vi "File_IO_Sample.vi"() -> ()   [LabVIEW 2025]
panel:
  out "Array 10":string[][](array[string])
  out "error out 2":errorcluster
  out "String 3":string
  out "Table Control":string[][](table)
  in  "Path":path
  out "error out":errorcluster
  in  "error in (no error)":errorcluster
  out "String 2":string
  in  "file path":path
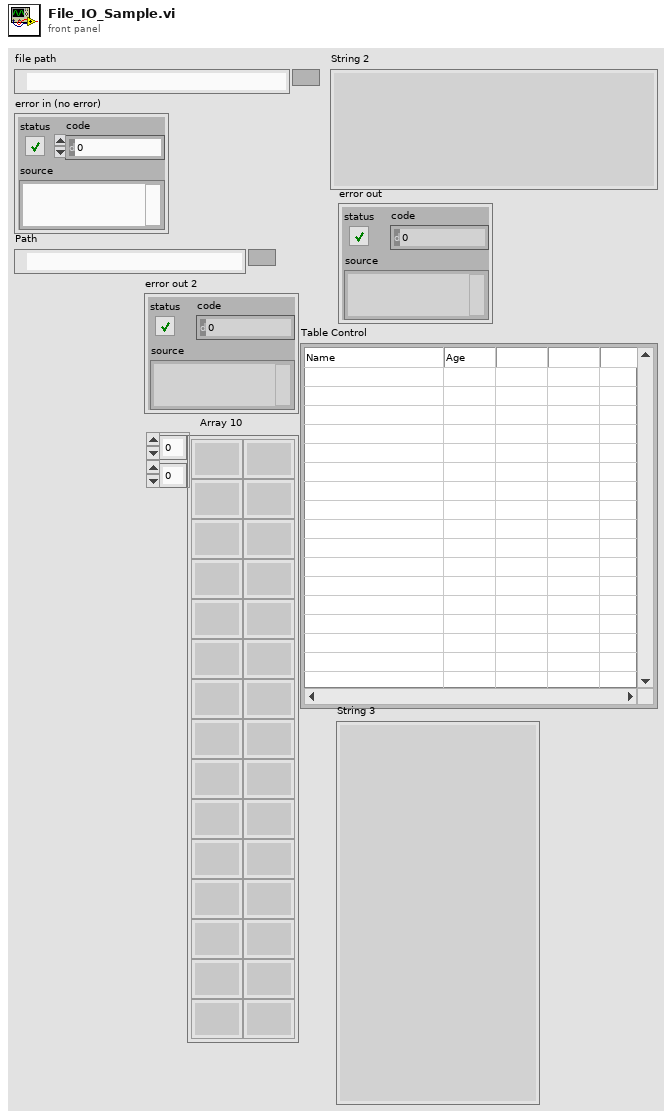
[diagram p1: front panel]
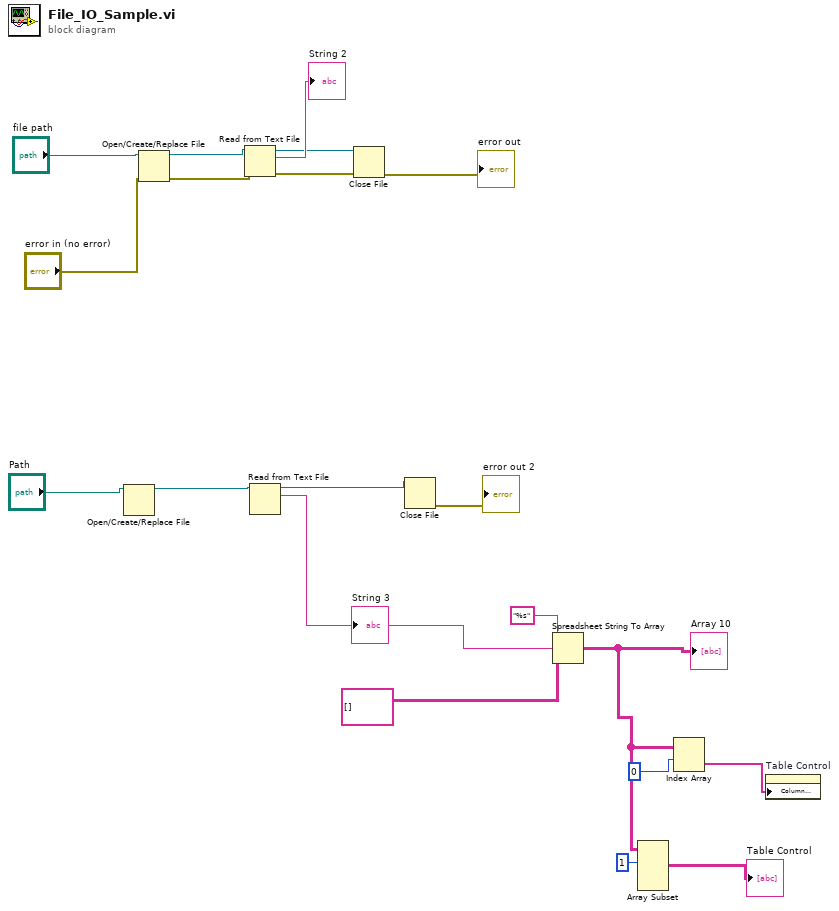
[diagram p0: block diagram]
diagram:
  n1 = Open/Create/Replace File(file path (use dialog)="Path") -> (refnum out=w11:refnum<file>)  [unwired: 5 in, 2 out]
  n2 = Open/Create/Replace File(file path (use dialog)="file path", error in="error in (no error)") -> (refnum out=w18:refnum<file>, error out=w17:errorcluster)  [unwired: 4 in, 1 out]
  n3 = Read from Text File(file (use dialog)=w18, error in=w17) -> (refnum out=w13:refnum<file>, text=→"String 2":string, error out=w15:errorcluster)  [unwired: 2 in, 1 out]
  n4 = Read from Text File(file (use dialog)=w11) -> (refnum out=w10:refnum<file>, text=w8:string)  [unwired: 3 in, 2 out]
  "String 3" <- w8
  n5 = Close File(refnum=w13, error in=w15) -> (error out=→"error out":errorcluster)  [unwired: 1 out]
  n6 = Close File(refnum=w10) -> (error out=→"error out 2":errorcluster)  [unwired: 1 in, 1 out]
  n7 = Spreadsheet String To Array(format string="%s", spreadsheet string=w8, array type (2D Dbl)=string[][] []) -> (array=w2:string[][])  [unwired: 1 in]
  "Array 10" <- w2
  n8 = Array Subset(array=w2, index (row)=1 ("index")) -> (→"Table Control":string[][])  [unwired: 3 in]
  n9 = Index Array(array=w2, index (row)=0) -> (element=w1:string[])  [unwired: 1 in]
  n10 = property on="Table Control" class="Tbl (strict)"("Column Headers[]"=w1) -> ()  [unwired: 2 in, 2 out]
